vi "Model 3566-Read Data.vi"(8 "error in":errorcluster) -> (0 "error out":errorcluster, 1 "Voltage":dbl, 2 "Resistance":dbl)   [LabVIEW 2018]
uses:
  Data Def/Model 3566-Setting.ctl
panel:
  out "Model 3566 Setting Out":T1
  in  "Model 3566 Setting In":T1
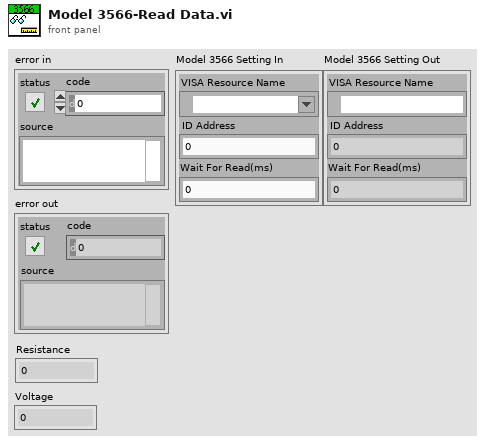
[diagram p1: front panel]
types:
  T1 = typedef "Model 3566-Setting.ctl" = cluster{"VISA Resource Name":refnum<visa-resource-name>, "ID Address":u8, "Wait For Read(ms)":u32}
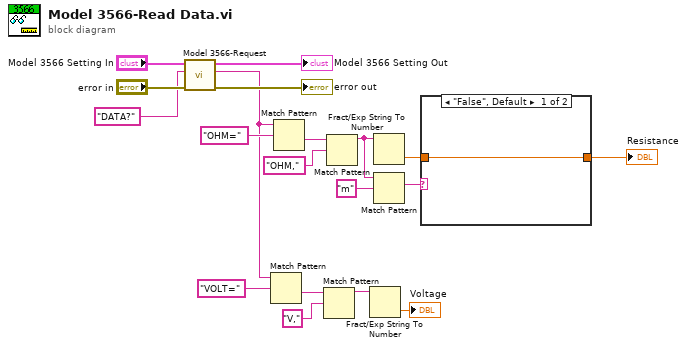
[diagram p0: block diagram]
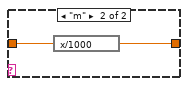
[diagram p2: hidden frame]
diagram:
  n1 = call "Model 3566-Request.vi"("error in"="error in", "Command"="DATA?" ("string"), "Model 3566 Setting In"="Model 3566 Setting In") -> ("error out"=→"error out":errorcluster, "Respond"=w10:string, "Model 3566 Setting Out"=→"Model 3566 Setting Out":T1)  [unwired: 6 in]
  n2 = Match Pattern(string=w10, regular expression="VOLT=") -> (after substring=w13:string)  [unwired: 1 in, 3 out]
  n3 = Match Pattern(string=w10, regular expression="OHM=") -> (after substring=w16:string)  [unwired: 1 in, 3 out]
  n4 = Match Pattern(string=w13, regular expression="V,") -> (before substring=w15:string)  [unwired: 1 in, 3 out]
  n5 = Match Pattern(string=w16, regular expression="OHM,") -> (before substring=w7:string)  [unwired: 1 in, 3 out]
  n6 = Fract/Exp String To Number(string=w15) -> (number=→"Voltage":dbl)  [unwired: 3 in, 1 out]
  n7 = Fract/Exp String To Number(string=w7) -> (number=w6:dbl)  [unwired: 3 in, 1 out]
  n8 = Match Pattern(string=w7, regular expression="m") -> (match substring=w3:string)  [unwired: 1 in, 3 out]
  n9 = case shown="\"False\", Default" w3 {
    tunnel: w6 -> [w20 w22]
    tunnel: [w20 w21] -> w5
    frame "False", Default {
    }
    frame "m" {
      n10 = expression code="x/1000"(w22) -> (w21:dbl)
    }
  }
  "Resistance" <- w5
